vi "Units_SecondsToMilliseconds.vi"(10 "Seconds":dbl) -> (2 "Milliseconds":dbl)   [LabVIEW 2019, in "Trajectory_Library.lvlib"]
doc: "Convert a value from seconds to milliseconds\n\nInputs: \n - Seconds\n\nOutputs:\n - Milliseconds"
uses:
  Trajectory_Library.lvlib
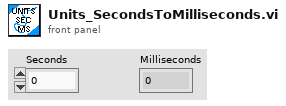
[diagram p1: front panel]
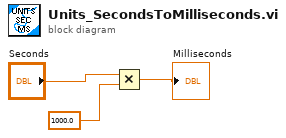
[diagram p0: block diagram]
diagram:
  n1 = Multiply(x="Seconds", y=1000.0) -> (x*y=→"Milliseconds":dbl)
